vi "Format Text.vi"(5 "Time Format String (%d/%m/%y %H:%M:%S%3u)":string="%d/%m/%y %H:%M:%S%3u", 7 "Debug Level":T1=enum."INFO", 8 "error in (no error)":errorcluster, 10 "Log Text":string, 11 "Logger in":refnum<class "Logger.lvclass">) -> (0 "error out":errorcluster, 1 "Log Output":string, 3 "Logger out":refnum<class "Logger.lvclass">)   [LabVIEW 2020, in "LV Logging.lvlib" / "Logger.lvclass"]
uses:
  Logger.lvclass
  Logger.lvclass/Logger.ctl
  Type Defs/Debug Level.ctl
  LV Logging.lvlib
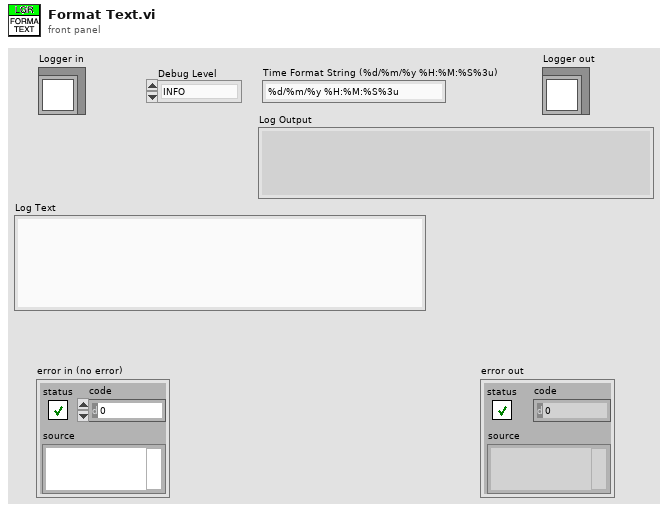
[diagram p1: front panel]
types:
  T1 = typedef "LV Logging.lvlib/Debug Level.ctl" = enum16{"DEBUG", "INFO", "WARN", "ERROR", "FATAL"}
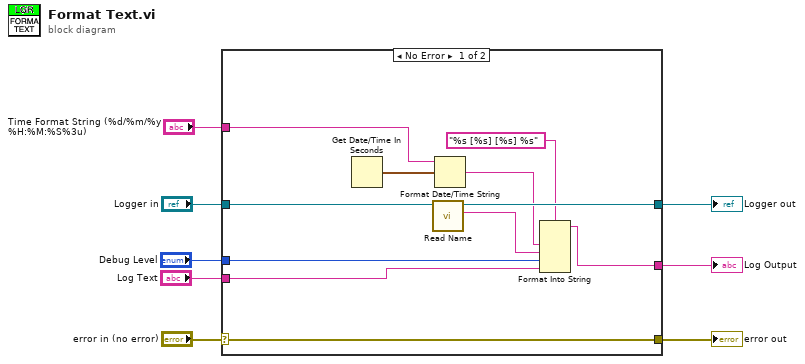
[diagram p0: block diagram]
diagram:
  n1 = case shown="No Error" "error in (no error)" {
    selector: "error in (no error)" -> [w19 w21]
    tunnel: [w19 w21] -> w6
    tunnel: [w17 w20] -> w5
    tunnel: "Logger in" -> [w18 w20]
    tunnel: "Log Text" -> [w15 _]
    tunnel: [w13 _] -> w3
    tunnel: "Debug Level" -> [w12 _]
    tunnel: "Time Format String (%d/%m/%y %H:%M:%S%3u)" -> [w9 _]
    frame No Error {
      n2 = Get Date/Time In Seconds() -> (seconds since 1Jan1904=w11:timestamp)
      n3 = call "Read Name.vi"("Logger in"=w18) -> ("Name"=w16:string, "Logger out"=w17:refnum<class "Logger.lvclass">)  [unwired: 8 in, 1 out]
      n4 = Format Date/Time String(time format string (%c)=w9, seconds (now)=w11) -> (date/time string=w10:string)  [unwired: 1 in]
      n5 = Format Into String(format string="%s [%s] [%s] %s", w10, w16, w12, w15) -> (resulting string=w13:string)  [unwired: 2 in, 1 out]
    }
    frame Error {
    }
  }
  "error out" <- w6
  "Logger out" <- w5
  "Log Output" <- w3
